vi "Shooter Control.vi"(11 "Time Delay Milli":dbl) -> ()   [LabVIEW 2011]
uses:
  System Set Points and States.vi
  <vilib>/addons/control/pid/pid.llb/PID (DBL).vi
  <vilib>/addons/control/pid/NI_PID_pid.lvlib
panel:
  out "RPM Error":cluster{dbl, dbl, dbl[]}(graph)
  out "Output 2":dbl
  out "Output":dbl
  out "Shooter Enabled":bool
  in  "Graph time interval  in seconds":dbl
  out "Shooter RPM":cluster{dbl, dbl, dbl[]}(graph)
  out "RPM Error":dbl
  out "Encoder Speed":dbl
  in  "D":dbl=0.001
  in  "I":dbl=0.05
  in  "P":dbl=0.001 step=0.001
  out "Encoder Set Speed":dbl
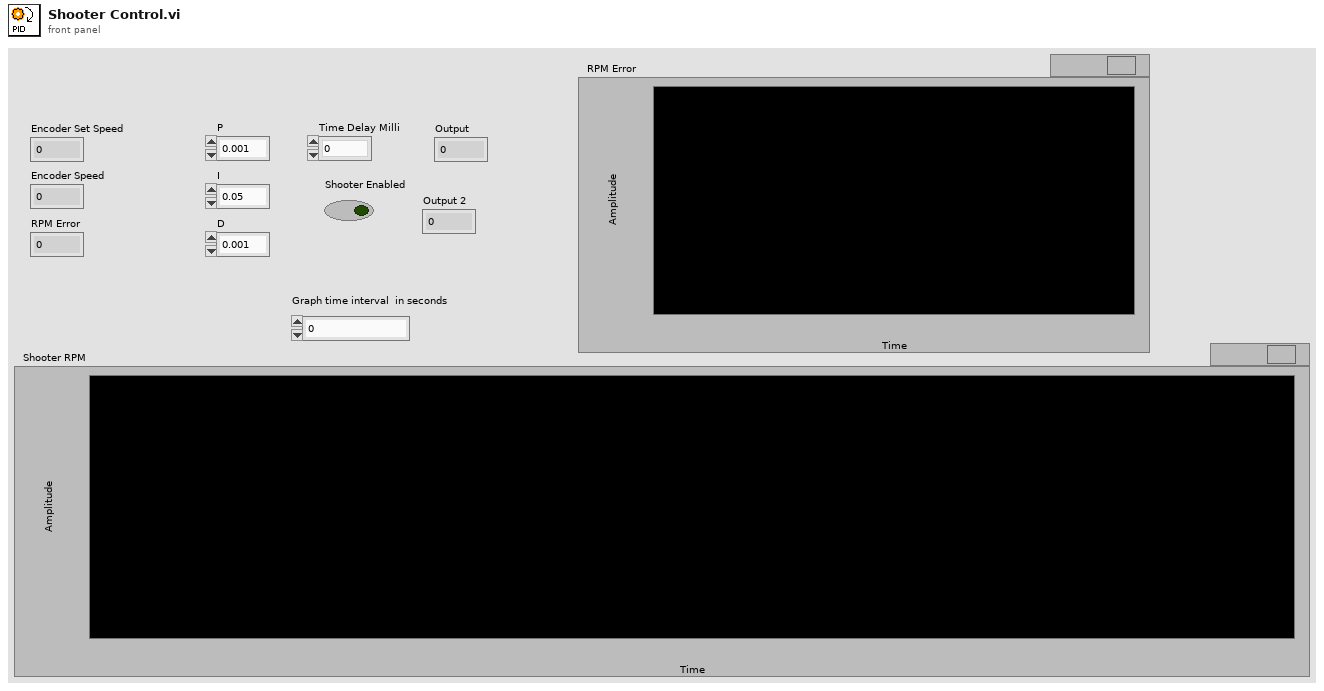
[diagram p1: front panel]
types:
  T1 = typedef "WPI_EncoderDevRef.ctl" = cluster{"DevStatus":errorcluster, "EncoderIndex":T2, "CounterIndex":T3, "DistancePerCount":dbl, "Decoding Type":T4}
  T2 = typedef "FPGA_EncoderIdx.ctl" = enum8{"Enc 0", "Enc 1", "Enc 2", "Enc 3", "Invalid"}
  T3 = typedef "FPGA_CounterCtrSystemIndex.ctl" = enum8{"Ctr 0", "Ctr 1", "Ctr 2", "Ctr 3", "Ctr 4", "Ctr 5", "Ctr 6", "Ctr 7", "Invalid"}
  T4 = typedef "WPI_EncoderType.ctl" = enum16{"1x", "2x", "4x"}
  T5 = typedef "WPI_MotorControlDeviceRef.ctl" = cluster{"DeviceStatus":errorcluster, "Type":enum16{"PWM", "CAN"}, "PWM":cluster{"Digital Module":T6, "PWM Channel":T7, "DeadBand":T8}, "CAN":cluster{"Device Number":u8, "Control Mode":T9, "Semaphore":T10, "Max Vout":dbl}, "Invert":bool, "TransformRef":T11, "InvTransformRef":T11}
  T6 = typedef "FPGA_TypedefDigitalModule.ctl" = enum16{"Digital Module 1", "Digital Module 2"}
  T7 = typedef "FPGA_DIOPWMChannel.ctl" = enum8{"PWM 1", "PWM 2", "PWM 3", "PWM 4", "PWM 5", "PWM 6", "PWM 7", "PWM 8", "PWM 9", "PWM 10", "Invalid"}
  T8 = typedef "WPI_PWMDeadband.ctl" = cluster{"Name":string, "maxPositivePwm":i32, "minPositivePwm":i32, "centerPwm":i32, "maxNegativePwm":i32, "minNegativePwm":i32, "angularRange":u16}
  T9 = typedef "WPI_CANJaguar_ControlMode.ctl" = enum8{"Percent VBus", "Current", "Speed", "Position", "Voltage"}
  T10 = typedef "Semaphore RefNum" = refnum<k1>
  T11 = typedef "WPI_PWMTransform_ConPane.ctl" = refnum<vi>
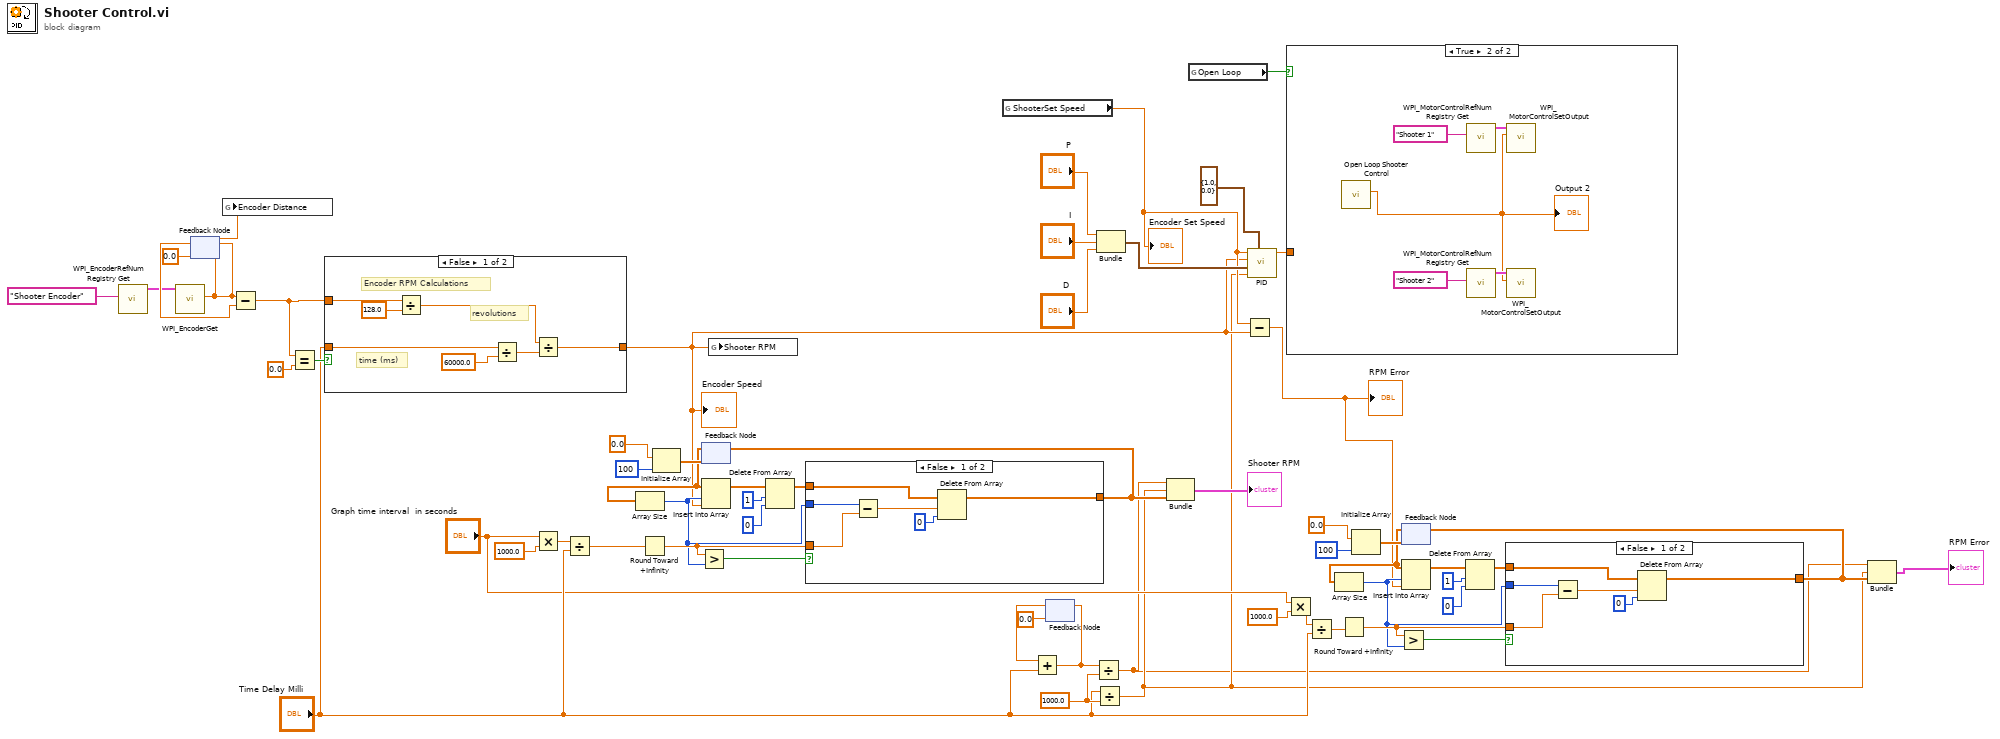
[diagram p0: block diagram]
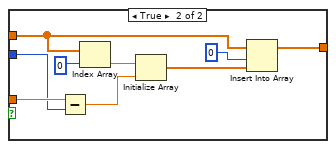
[diagram p2: hidden frame]
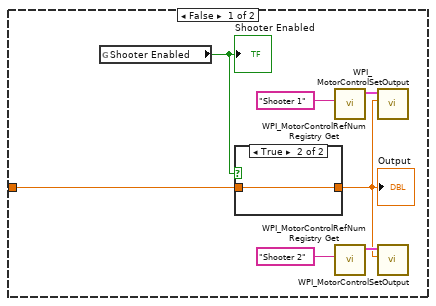
[diagram p3: hidden frame]
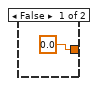
[diagram p4: hidden frame]
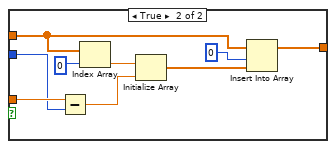
[diagram p5: hidden frame]
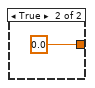
[diagram p6: hidden frame]
diagram:
  w36 = 1000.0 ("y")
  n1 = call <vilib>:"WPI_EncoderRefNum Registry Get.vi"("refnum name"="Shooter Encoder") -> ("EncoderDevRef"=w44:T1)  [unwired: 9 in, 1 out]
  n2 = call <vilib>:"WPI_EncoderGet.vi"("EncoderDevRef"=w44) -> ("Distance"=w22:dbl)  [unwired: 5 in, 5 out]
  n3 = feedback #1(0.0) -> (w50:dbl)
  n4 = feedback-in #1(w22) -> ()
  n5 = global write "System Set Points and States.vi" "Encoder Distance"(w22) -> ()
  n6 = Subtract(x=w22, y=w50) -> (x-y=w23:dbl)
  n7 = Equal?(x=w23, y=0.0) -> (x = y?=w46:bool)
  n8 = case shown="False" w46 {
    tunnel: [w65 0.0] -> w26
    tunnel: w23 -> [w64 _]
    tunnel: "Time Delay Milli" -> [w62 _]
    frame False {
      # "time (ms)"
      # "revolutions"
      # "Encoder RPM Calculations"
      n9 = Divide(x=w64, y=128.0) -> (x/y=w63:dbl)
      n10 = Divide(x=w62, y=60000.0) -> (x/y=w60:dbl)
      n11 = Divide(x=w63, y=w60) -> (x/y=w65:dbl)
    }
    frame True {
    }
  }
  "Encoder Speed" <- w26
  n12 = Multiply(x="Graph time interval  in seconds", y=1000.0) -> (x*y=w33:dbl)
  n13 = Divide(x=w33, y="Time Delay Milli") -> (x/y=w32:dbl)
  n14 = Round Toward +Infinity(x=w32) -> (ceil(x): smallest int >= x=w29:dbl)
  n15 = Initialize Array(0.0 ("element"), 100 ("dimension size")) -> (w52:dbl[])
  n16 = feedback #2(w52) -> (w42:dbl[])
  n17 = Array Size(array=w42) -> (size(s)=w28:i32)
  n18 = Greater?(x=w29, y=w28) -> (0:w31:bool)
  n19 = Insert Into Array(array=w42, index=w28, new element=w26) -> (w41:dbl[])
  n20 = global write "System Set Points and States.vi" "Shooter RPM"(w26) -> ()
  n21 = Delete From Array(array=w41, length=1, index=0) -> (array with subset deleted=w30:dbl[])  [unwired: 1 out]
  n22 = case shown="False" w31 {
    tunnel: w30 -> [w68 w80]
    tunnel: w29 -> [w70 w78]
    tunnel: w28 -> [w71 w77]
    tunnel: [w67 w73] -> w27
    frame False {
      n23 = Subtract(x=w71, y=w70) -> (x-y=w69:dbl)
      n24 = Delete From Array(array=w68, length=w69, index=0) -> (array with subset deleted=w67:dbl[])  [unwired: 1 out]
    }
    frame True {
      n25 = Subtract(x=w78, y=w77) -> (x-y=w76:dbl)
      n26 = Index Array(array=w80, index=0) -> (element=w81:dbl)
      n27 = Initialize Array(w81, w76) -> (w75:dbl[])
      n28 = Insert Into Array(array=w80, index=0, new element=w75) -> (w73:dbl[])
    }
  }
  n29 = feedback-in #2(w27) -> ()
  n30 = global read "System Set Points and States.vi" "ShooterSet Speed"() -> (w53:dbl)
  "Encoder Set Speed" <- w53
  n31 = feedback #3(0.0) -> (w37:dbl)
  n32 = Add(x=w37, y="Time Delay Milli") -> (x+y=w35:dbl)
  n33 = feedback-in #3(w35) -> ()
  n34 = Divide(x=w35, y=w36) -> (x/y=w2:dbl)
  n35 = Divide(x="Time Delay Milli", y=w36) -> (x/y=w3:dbl)
  n36 = Bundle("P"="P", "I"="I", "D"="D") -> (w54:cluster{"P":dbl, "I":dbl, "D":dbl})  [unwired: 1 in]
  n37 = Bundle(w2, w3, w27) -> (→"Shooter RPM":cluster{dbl, dbl, dbl[]})  [unwired: 1 in]
  n38 = global read "System Set Points and States.vi" "Open Loop"() -> (w24:bool)
  n39 = Subtract(x=w53, y=w26) -> (x-y=w5:dbl)
  "RPM Error" <- w5
  n40 = call-poly <vilib>:"PID.vi"("output range"=cluster{"output high":dbl, "output low":dbl} {"output high"=1.0, "output low"=0.0}, "dt (s)"=w3, "PID gains"=w54, "process variable"=w26, "setpoint"=w53) -> ("output"=w25:dbl)  [unwired: 5 in, 1 out]
  n41 = case shown="True" w24 {
    tunnel: w25 -> [w84 _]
    frame False {
      n42 = global read "System Set Points and States.vi" "Shooter Enabled"() -> (w83:bool)
      "Shooter Enabled" <- w83
      n43 = case shown="True" w83 {
        tunnel: w84 -> [_ w90]
        tunnel: [0.0 ("output") w90] -> w82
        frame False {
        }
        frame True {
        }
      }
      "Output" <- w82
      n44 = call <vilib>:"WPI_MotorControlRefNum Registry Get.vi"("refnum name"="Shooter 1") -> ("MotorControlDevRef"=w87:T5)  [unwired: 9 in, 1 out]
      n45 = call <vilib>:"WPI_MotorControlRefNum Registry Get.vi"("refnum name"="Shooter 2") -> ("MotorControlDevRef"=w86:T5)  [unwired: 9 in, 1 out]
      n46 = call <vilib>:"WPI_MotorControlSetOutput.vi"("Output"=w82, "MotorControlDevRef"=w87) -> ()  [unwired: 8 in, 2 out]
      n47 = call <vilib>:"WPI_MotorControlSetOutput.vi"("Output"=w82, "MotorControlDevRef"=w86) -> ()  [unwired: 8 in, 2 out]
    }
    frame True {
      n48 = call "Open Loop Shooter Control.vi"() -> ("Open Loop PWM"=w91:dbl)  [unwired: 11 in]
      "Output 2" <- w91
      n49 = call <vilib>:"WPI_MotorControlRefNum Registry Get.vi"("refnum name"="Shooter 1") -> ("MotorControlDevRef"=w94:T5)  [unwired: 9 in, 1 out]
      n50 = call <vilib>:"WPI_MotorControlRefNum Registry Get.vi"("refnum name"="Shooter 2") -> ("MotorControlDevRef"=w93:T5)  [unwired: 9 in, 1 out]
      n51 = call <vilib>:"WPI_MotorControlSetOutput.vi"("Output"=w91, "MotorControlDevRef"=w94) -> ()  [unwired: 8 in, 2 out]
      n52 = call <vilib>:"WPI_MotorControlSetOutput.vi"("Output"=w91, "MotorControlDevRef"=w93) -> ()  [unwired: 8 in, 2 out]
    }
  }
  n53 = Multiply(x="Graph time interval  in seconds", y=1000.0) -> (x*y=w8:dbl)
  n54 = Divide(x=w8, y="Time Delay Milli") -> (x/y=w11:dbl)
  n55 = Round Toward +Infinity(x=w11) -> (ceil(x): smallest int >= x=w13:dbl)
  n56 = Initialize Array(0.0 ("element"), 100 ("dimension size")) -> (w21:dbl[])
  n57 = feedback #4(w21) -> (w10:dbl[])
  n58 = Array Size(array=w10) -> (size(s)=w12:i32)
  n59 = Greater?(x=w13, y=w12) -> (0:w15:bool)
  n60 = Insert Into Array(array=w10, index=w12, new element=w5) -> (w18:dbl[])
  n61 = Delete From Array(array=w18, length=1, index=0) -> (array with subset deleted=w14:dbl[])  [unwired: 1 out]
  n62 = case shown="False" w15 {
    tunnel: w14 -> [w97 w109]
    tunnel: w13 -> [w99 w107]
    tunnel: w12 -> [w100 w106]
    tunnel: [w96 w102] -> w4
    frame False {
      n63 = Subtract(x=w100, y=w99) -> (x-y=w98:dbl)
      n64 = Delete From Array(array=w97, length=w98, index=0) -> (array with subset deleted=w96:dbl[])  [unwired: 1 out]
    }
    frame True {
      n65 = Subtract(x=w107, y=w106) -> (x-y=w105:dbl)
      n66 = Index Array(array=w109, index=0) -> (element=w110:dbl)
      n67 = Initialize Array(w110, w105) -> (w104:dbl[])
      n68 = Insert Into Array(array=w109, index=0, new element=w104) -> (w102:dbl[])
    }
  }
  n69 = feedback-in #4(w4) -> ()
  n70 = Bundle(w2, w3, w4) -> (→"RPM Error":cluster{dbl, dbl, dbl[]})  [unwired: 1 in]
